vi "Set Rotation.vi"(8 "error in (no error)":errorcluster, 9 "Angle":sgl, 10 "Axis":cluster{"X":sgl, "Y":sgl, "Z":sgl}, 11 "Scene Object":refnum<vi>) -> (0 "error out":errorcluster, 3 "Rotated Scene Object":refnum<vi>)   [LabVIEW 2020, in "NI_3D Picture Control.lvlib"]
doc: "Clears any rotations previously applied to an object in a 3D scene and rotates the object by the values <B>Axis</B> and <B>Angle</B>. This VI performs an absolute rotation from the object's initial position."
uses:
  <vilib>/picture/3D Picture Control/NI_3D Picture Control.lvlib
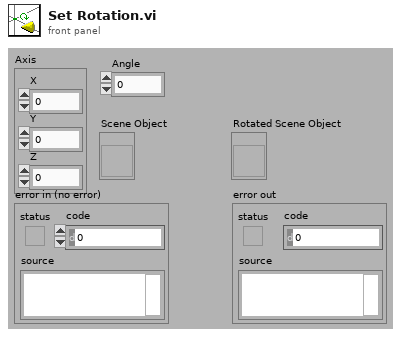
[diagram p1: front panel]
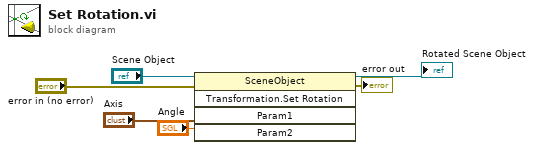
[diagram p0: block diagram]
diagram:
  n1 = invoke class="SceneObject" method="Transformation.Set Rotation"(reference="Scene Object", error in="error in (no error)", "Param1"="Axis", "Param2"="Angle") -> (reference out=→"Rotated Scene Object":refnum<vi>, error out=→"error out":errorcluster)  [unwired: 1 in, 3 out]
